vi "Init Plugin.vi"(8 "error in (no error)":errorcluster, 11 "object in":refnum<class "UserInfoManageUI.lvclass">) -> (0 "error out":errorcluster, 3 "object out":refnum<class "UserInfoManageUI.lvclass">)   [LabVIEW 2015]
doc: "Functions : <b> 1. check if table has been built;\n 2. set ID auto Increment and primary key\n 3. set 简介 to long text"
uses:
  Plugin/Plugin.lvclass
  DatabaseManagement/Database.lvclass
  UserInfoManageUI.lvclass
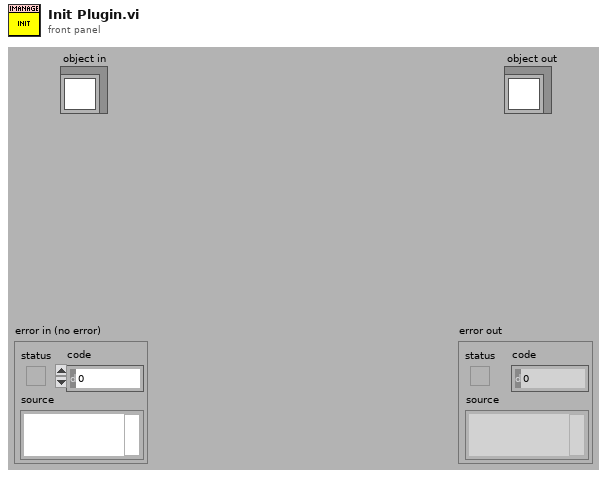
[diagram p1: front panel]
types:
  T1 = typedef "NI_Database_API.lvlib/DB Tools Column Info.ctl" = cluster{"column name":string, "data type":T2, "size":i32, "allow null?":bool}
  T2 = typedef "NI_Database_API.lvlib/DB Tools DataTypes.ctl" = enum16{"String", "Long (I32)", "Single (SGL)", "Double (DBL)", "Date/Time", "Binary"}
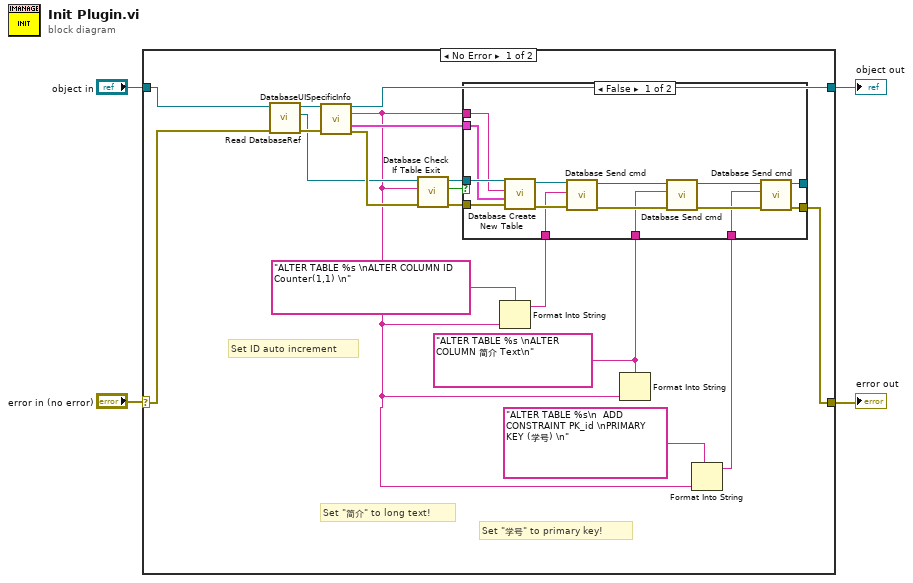
[diagram p0: block diagram]
diagram:
  n1 = case shown="No Error" "error in (no error)" {
    selector: "error in (no error)" -> [w10 w40]
    tunnel: "object in" -> [w11 w41]
    tunnel: [w17 w41] -> w3
    tunnel: [w14 w40] -> w1
    frame No Error {
      w9 = "ALTER TABLE %s \nALTER COLUMN 简介 Text\n" ("SQL query")
      # "Set \"学号\" to primary key!"
      # "Set \"简介\" to long text!"
      # "Set ID auto increment"
      n2 = call "Read DatabaseRef.vi"("error in (no error)"=w10, "Plugin in"=w11) -> ("error out"=w18:errorcluster, "Database.lvlib:Database"=w13:refnum<class "Database.lvclass">, "Plugin out"=w19:refnum<class "UserInfoManageUI.lvclass">)  [unwired: 7 in]
      n3 = call-dynamic "DatabaseUISpecificInfo.vi"("UserInfoManage"=w19, "error in (no error)"=w18) -> ("UserInfoManage out"=w17:refnum<class "UserInfoManageUI.lvclass">, "TableName"=w5:string, "column information"=w15:T1[], "error out"=w16:errorcluster)  [unwired: 9 in, 1 out]
      n4 = call "Database Check If Table Exit.vi"("error in (no error)"=w16, "Table"=w5, "Database in"=w13) -> ("error out"=w20:errorcluster, "Exit?"=w22:bool, "Database out"=w21:refnum<class "Database.lvclass">)  [unwired: 6 in]
      n5 = Format Into String(format string="ALTER TABLE %s \nALTER COLUMN ID Counter(1,1) \n" ("SQL query"), w5) -> (resulting string=w7:string)  [unwired: 2 in, 1 out]
      n6 = Format Into String(format string=w9, w5) -> ()  [unwired: 2 in, 2 out]
      n7 = Format Into String(format string="ALTER TABLE %s\n  ADD CONSTRAINT PK_id \nPRIMARY KEY (学号) \n" ("SQL query"), w5) -> (resulting string=w6:string)  [unwired: 2 in, 1 out]
      n8 = case shown="False" w22 {
        tunnel: w21 -> [w37 w38]
        tunnel: w20 -> [w36 w39]
        tunnel: w15 -> [w35 _]
        tunnel: w5 -> [w34 _]
        tunnel: [w25 w39] -> w14
        tunnel: [w26 w38] -> _
        tunnel: w9 -> [w29 _]
        tunnel: w7 -> [w24 _]
        tunnel: w6 -> [w23 _]
        frame False {
          n9 = call "Database Create New Table.vi"("error in (no error)"=w36, "column information"=w35, "table"=w34, "Database in"=w37) -> ("error out"=w32:errorcluster, "Database out"=w33:refnum<class "Database.lvclass">)  [unwired: 6 in]
          n10 = call "Database Send cmd.vi"("error in (no error)"=w32, "SQL query"=w24, "Database in"=w33) -> ("error out"=w30:errorcluster, "Database out"=w31:refnum<class "Database.lvclass">)  [unwired: 7 in]
          n11 = call "Database Send cmd.vi"("error in (no error)"=w30, "SQL query"=w29, "Database in"=w31) -> ("error out"=w27:errorcluster, "Database out"=w28:refnum<class "Database.lvclass">)  [unwired: 7 in]
          n12 = call "Database Send cmd.vi"("error in (no error)"=w27, "SQL query"=w23, "Database in"=w28) -> ("error out"=w25:errorcluster, "Database out"=w26:refnum<class "Database.lvclass">)  [unwired: 7 in]
        }
        frame True {
        }
      }
    }
    frame Error {
    }
  }
  "object out" <- w3
  "error out" <- w1
